vi "Zero Global.vi"() -> ()   [LabVIEW 2017, in "NI_Gmath.lvlib"]
uses:
  NI_Gmath.lvlib
panel:
  in  "list of variables":i32[](array[numeric])=[0, 0]
  in  "time":string="t"
  in  "X":string[](array[string])=["x1", "x2"]
  out "result":dbl[][](array[numeric]) format="%.2f"
  out "table":i32[][][](array[numeric])
  # "operator"
  # "register1"
  # "register2"
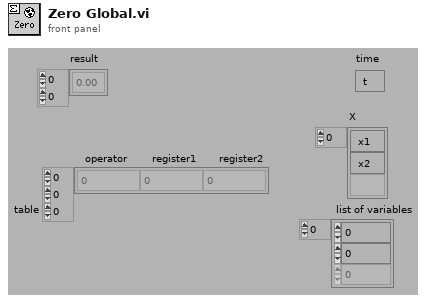
[diagram p1: front panel]
diagram:
